vi "Q_Get Total Distance by day grouped by team.vi"(8 "error in (no error)":errorcluster, 10 "current time":timestamp, 11 "Data Manager in":refnum<class "Data Manager.lvclass">) -> (0 "error out":errorcluster, 1 "Group B Daily":dbl, 2 "Group A Daily":dbl, 3 "Data Manager out":refnum<class "Data Manager.lvclass">)   [LabVIEW 2020, in "Data Manager.lvclass"]
uses:
  Data Manager.lvclass
  Data Manager.lvclass/Data Manager.ctl
  <vilib>/drjdpowell/SQLite Library/SQL Connection/Execute SQL.vi
  <vilib>/drjdpowell/SQLite Library/SQLite.lvlib
  <vilib>/addons/_JKI.lib/Serialization/JSON/Serializer/JSON Serializer/JSON Serializer.lvclass
  <vilib>/drjdpowell/SQLite Library/SQL Connection/Connection.lvclass
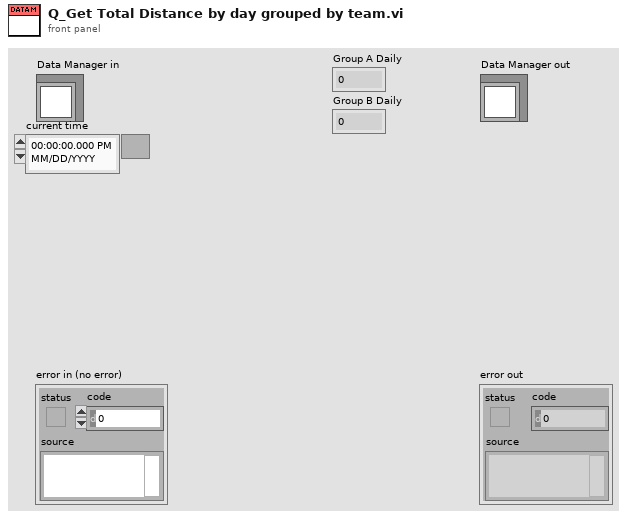
[diagram p1: front panel]
types:
  T1 = typedef "LVDateTimeRec.ctl" = cluster{"fractional second":dbl, "second":i32, "minute":i32, "hour":i32, "day of month":i32, "month":i32, "year":i32, "day of week":i32, "day of year":i32, "DST":i32}
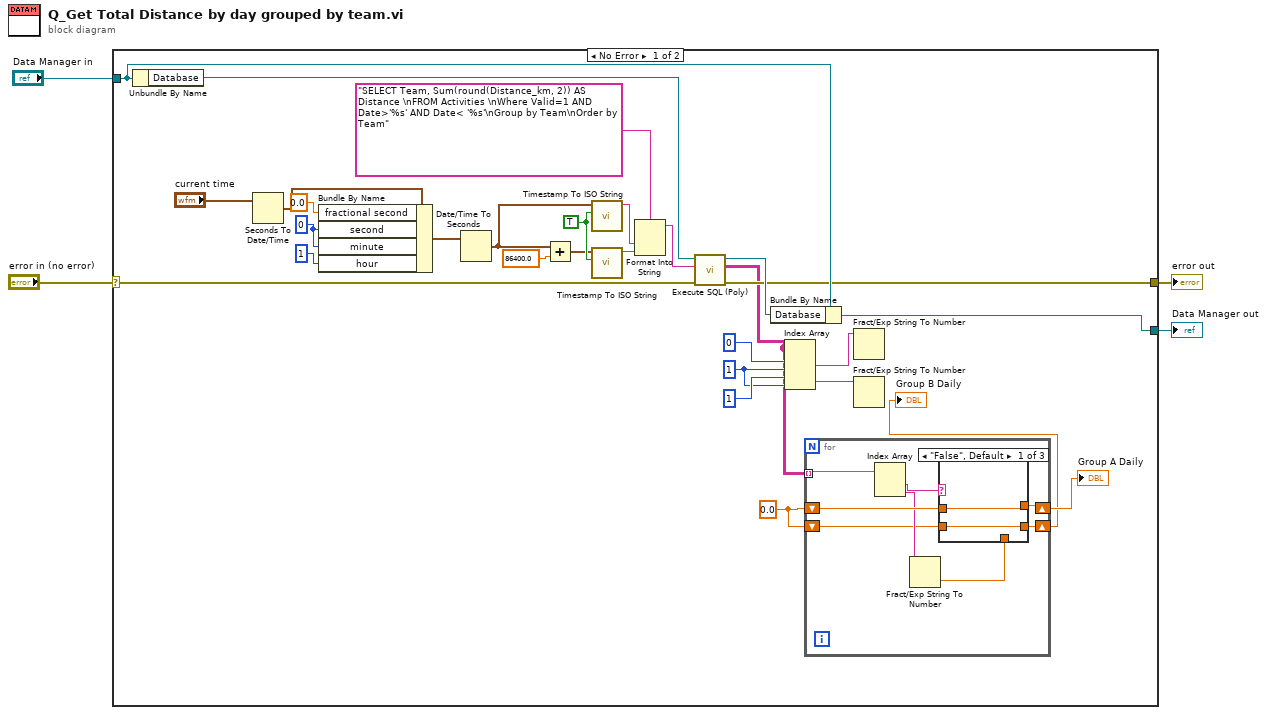
[diagram p0: block diagram]
diagram:
  n1 = case shown="No Error" "error in (no error)" {
    selector: "error in (no error)" -> [w29 w49]
    tunnel: [w28 w49] -> w3
    tunnel: [w31 w48] -> w1
    tunnel: "Data Manager in" -> [w32 w48]
    frame No Error {
      w7 = 0.0
      w12 = 1 ("disabled index (col)")
      w20 = TRUE ("Universal time (F)")
      w23 = 0 ("minute")
      n2 = Unbundle By Name(w32) -> ("Database"=w33:refnum<class "Connection.lvclass">)
      n3 = Seconds To Date/Time(time stamp (now)="current time") -> (date time rec=w26:T1)  [unwired: 1 in]
      n4 = Bundle By Name(cluster=w26, "fractional second"=0.0, "second"=w23, "minute"=w23, "hour"=1) -> (w27:T1)
      n5 = Date/Time To Seconds(2:w27) -> (0:w21:timestamp)  [unwired: 1 in]
      n6 = Add(x=w21, y=86400.0) -> (x+y=w19:timestamp)
      n7 = call <vilib>:"Timestamp To ISO String.vi"("Universal time (F)"=w20, "Timestamp"=w21) -> ("ISO Timestamp String"=w17:string)  [unwired: 8 in, 1 out]
      n8 = call <vilib>:"Timestamp To ISO String.vi"("Universal time (F)"=w20, "Timestamp"=w19) -> ("ISO Timestamp String"=w16:string)  [unwired: 8 in, 1 out]
      n9 = Format Into String(format string="SELECT Team, Sum(round(Distance_km, 2)) AS Distance \nFROM Activities \nWhere Valid=1 AND Date>'%s' AND Date< '%s'\nGroup by Team\nOrder by Team" ("SQL"), w17, w16) -> (resulting string=w15:string)  [unwired: 2 in, 1 out]
      n10 = call-poly <vilib>:"Execute SQL (Poly).vi"("error in (no error)"=w29, "SQL"=w15, "SQLite Connection in"=w33) -> ("error out"=w28:errorcluster, "Result Set"=w8:string[][], "SQLite Connection"=w30:refnum<class "Connection.lvclass">)  [unwired: 5 in, 1 out]
      n11 = Bundle By Name(cluster=w32, "Database"=w30) -> (w31:refnum<class "Data Manager.lvclass">)
      n12 = Index Array(array=w8, index (row) #1=0 ("index (row)"), index (col) #1=w12, index (row) #2=1 ("index (row)"), index (col) #2=w12) -> (element #1=w10:string, element #2=w11:string)
      n13 = for {
        tunnel: w8 -> [w41] mode=indexing
        shift-right: [w37] -> w6
        shift-left: w7 -> [w39]
        shift-right: [w34] -> w5
        shift-left: w7 -> [w35]
        n14 = Index Array(array=w41) -> (element #1=w40:string, element #2=w38:string)  [unwired: 2 in]
        n15 = Fract/Exp String To Number(string=w38) -> (number=w36:dbl)  [unwired: 3 in, 1 out]
        n16 = case shown="\"False\", Default" w40 {
          tunnel: w39 -> [w43 _ w47]
          tunnel: [w43 w45 w47] -> w37
          tunnel: w36 -> [_ w45 w46]
          tunnel: w35 -> [w42 w44 _]
          tunnel: [w42 w44 w46] -> w34
          frame "False", Default {
          }
          frame "Group A" {
          }
          frame "Group B" {
          }
        }
      }
      "Group A Daily" <- w6
      "Group B Daily" <- w5
      n17 = Fract/Exp String To Number(string=w10) -> ()  [unwired: 3 in, 2 out]
      n18 = Fract/Exp String To Number(string=w11) -> ()  [unwired: 3 in, 2 out]
    }
    frame Error {
    }
  }
  "error out" <- w3
  "Data Manager out" <- w1
